vi "background writer.vi"(1 "command queue":refnum<k33>, 2 "response from processor":refnum<k33>, 3 "output type order":T6[](array[typedef]), 5 "dictionary":T4, 7 "Ring Buffer":T1, 9 "cache allocation":T5, 11 "Logging Configuration":T2={"logging path"=path "", "backup directory"=path "", "group name"="", "scans per write"=20, "has enable channel"=FALSE, "enable channel (bool)"=0, "has trigger channel"=FALSE, "trigger channel (bool)"=0, "Blocks to log"=0, "Pre-trigger samples?"=FALSE, "Edge Direction"=enum."Rising", "LogRotate"=refnum}) -> (15 "error out":errorcluster)   [LabVIEW 2015, in "TDMS datalogger runtime.lvclass"]
uses:
  TDMS datalogger runtime.lvclass
  <vilib>/NI/Tag Bus/tag/Data Type.ctl
  data cache.ctl
  <vilib>/NI/Tag Bus/dictionary/full data dictionary.ctl
  message to background process.ctl
  control enum.ctl
  <vilib>/NI/Tag Bus/table/data table.ctl
  response from background process.ctl
  response enum.ctl
  Logging Configuration.ctl
  <vilib>/NI/LogRotate/LogRotate.lvclass
  configuration/Edge Direction.ctl
  Ring Buffer.ctl
  writer state enum.ctl
  <vilib>/NI/Tag Bus/table/data table.lvlib
  <vilib>/NI/Tag Bus/tag/tag descriptor.lvclass
  <vilib>/NI/Tag Bus/dictionary/data dictionary.lvclass
  configuration/TDMS datalogger configuration.lvclass
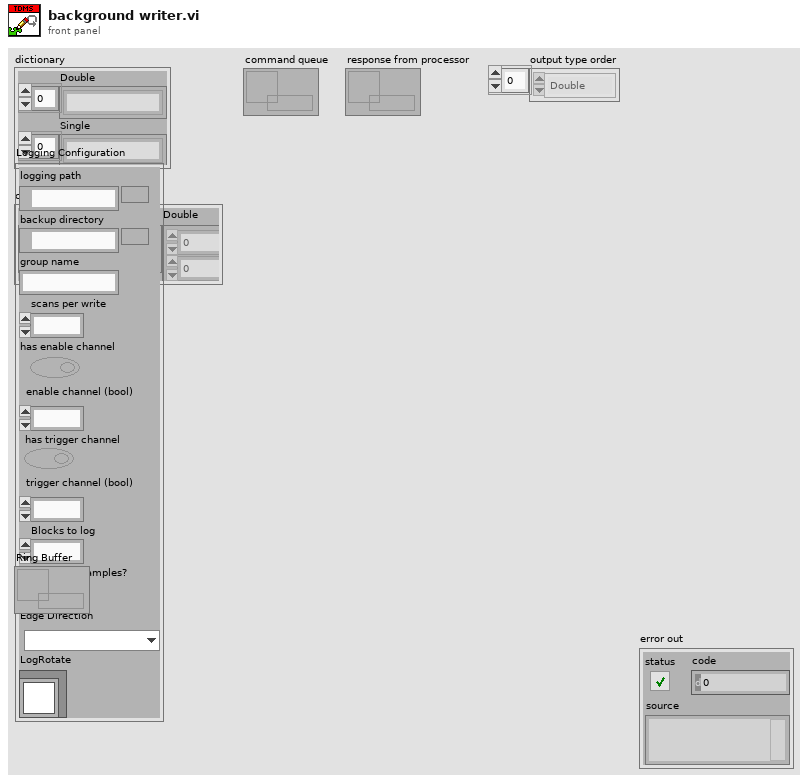
[diagram p1: front panel]
types:
  T1 = typedef "TDMS datalogger runtime.lvclass/Ring Buffer.ctl" = refnum<queue>
  T2 = typedef "TDMS datalogger runtime.lvclass/Logging Configuration.ctl" = cluster{"logging path":path, "backup directory":path, "group name":string, "scans per write":u16, "has enable channel":bool, "enable channel (bool)":i32, "has trigger channel":bool, "trigger channel (bool)":i32, "Blocks to log":i32, "Pre-trigger samples?":bool, "Edge Direction":T3, "LogRotate":refnum<class "LogRotate.lvclass">}
  T3 = typedef "TDMS datalogger configuration.lvclass/Edge Direction.ctl" = enum16{"Rising", "Falling"}
  T4 = typedef "tag bus.lvlib/data dictionary.lvclass/full data dictionary.ctl" = cluster{"Double":string[], "Single":string[], "I64":string[], "I32":string[], "I16":string[], "I8":string[], "U64":string[], "U32":string[], "U16":string[], "U8":string[], "Boolean":string[], "String":string[], "Array of Double":string[], "Array of Single":string[], "Array of I64":string[], "Array of I32":string[], "Array of I16":string[], "Array of I8":string[], "Array of U64":string[], "Array of U32":string[], "Array of U16":string[], "Array of U8":string[], "Array of Boolean":string[], "Array of String":string[]}
  T5 = typedef "TDMS datalogger runtime.lvclass/data cache.ctl" = cluster{"timestamps":timestamp[], "Double":dbl[][], "Single":sgl[][], "I64":i64[][], "I32":i32[][], "I16":i16[][], "I8":i8[][], "U64":u64[][], "U32":u32[][], "U16":u16[][], "U8":u8[][], "Boolean":bool[][]}
  T6 = typedef "tag bus.lvlib/tag descriptor.lvclass/Data Type.ctl" = enum16{"Double", "Single", "I64", "I32", "I16", "I8", "U64", "U32", "U16", "U8", "Boolean", "String", "Array of Double", "Array of Single", "Array of I64", "Array of I32", "Array of I16", "Array of I8", "Array of U64", "Array of U32", "Array of U16", "Array of U8", "Array of Boolean", "Array of String"}
  T7 = typedef "TDMS datalogger runtime.lvclass/writer state enum.ctl" = enum16{"wait for message", "create file", "report error", "exit", "close file"}
  T8 = typedef "TDMS datalogger runtime.lvclass/response enum.ctl" = enum16{"exit", "return buffer", "error"}
  T9 = typedef "TDMS datalogger runtime.lvclass/response from background process.ctl" = cluster{"response enum":T8, "datapack":refnum<data-value>, "error code":i32}
  T10 = typedef "TDMS datalogger runtime.lvclass/message to background process.ctl" = cluster{"control enum":T11, "datapack":refnum<data-value>, "Time Stamp":timestamp}
  T11 = typedef "TDMS datalogger runtime.lvclass/control enum.ctl" = enum16{"exit", "output data"}
  T12 = typedef "tag bus.lvlib/data table.lvlib/data table.ctl" = cluster{"Double":dbl[], "Single":sgl[], "I64":i64[], "I32":i32[], "I16":i16[], "I8":i8[], "U64":u64[], "U32":u32[], "U16":u16[], "U8":u8[], "Boolean":bool[], "String":string[], "Array of Double":cluster{"DBL Array":dbl[]}[], "Array of Single":cluster{"SGL Array":sgl[]}[], "Array of I64":cluster{"I64 Array":i64[]}[], "Array of I32":cluster{"I32 Array":i32[]}[], "Array of I16":cluster{"I16 Array":i16[]}[], "Array of I8":cluster{"I8 Array":i8[]}[], "Array of U64":cluster{"U64 Array":u64[]}[], "Array of U32":cluster{"U32 Array":u32[]}[], "Array of U16":cluster{"U16 Array":u16[]}[], "Array of U8":cluster{"U8 Array":u8[]}[], "Array of Boolean":cluster{"Boolean Array":bool[]}[], "Array of String":cluster{"String Array":string[]}[]}
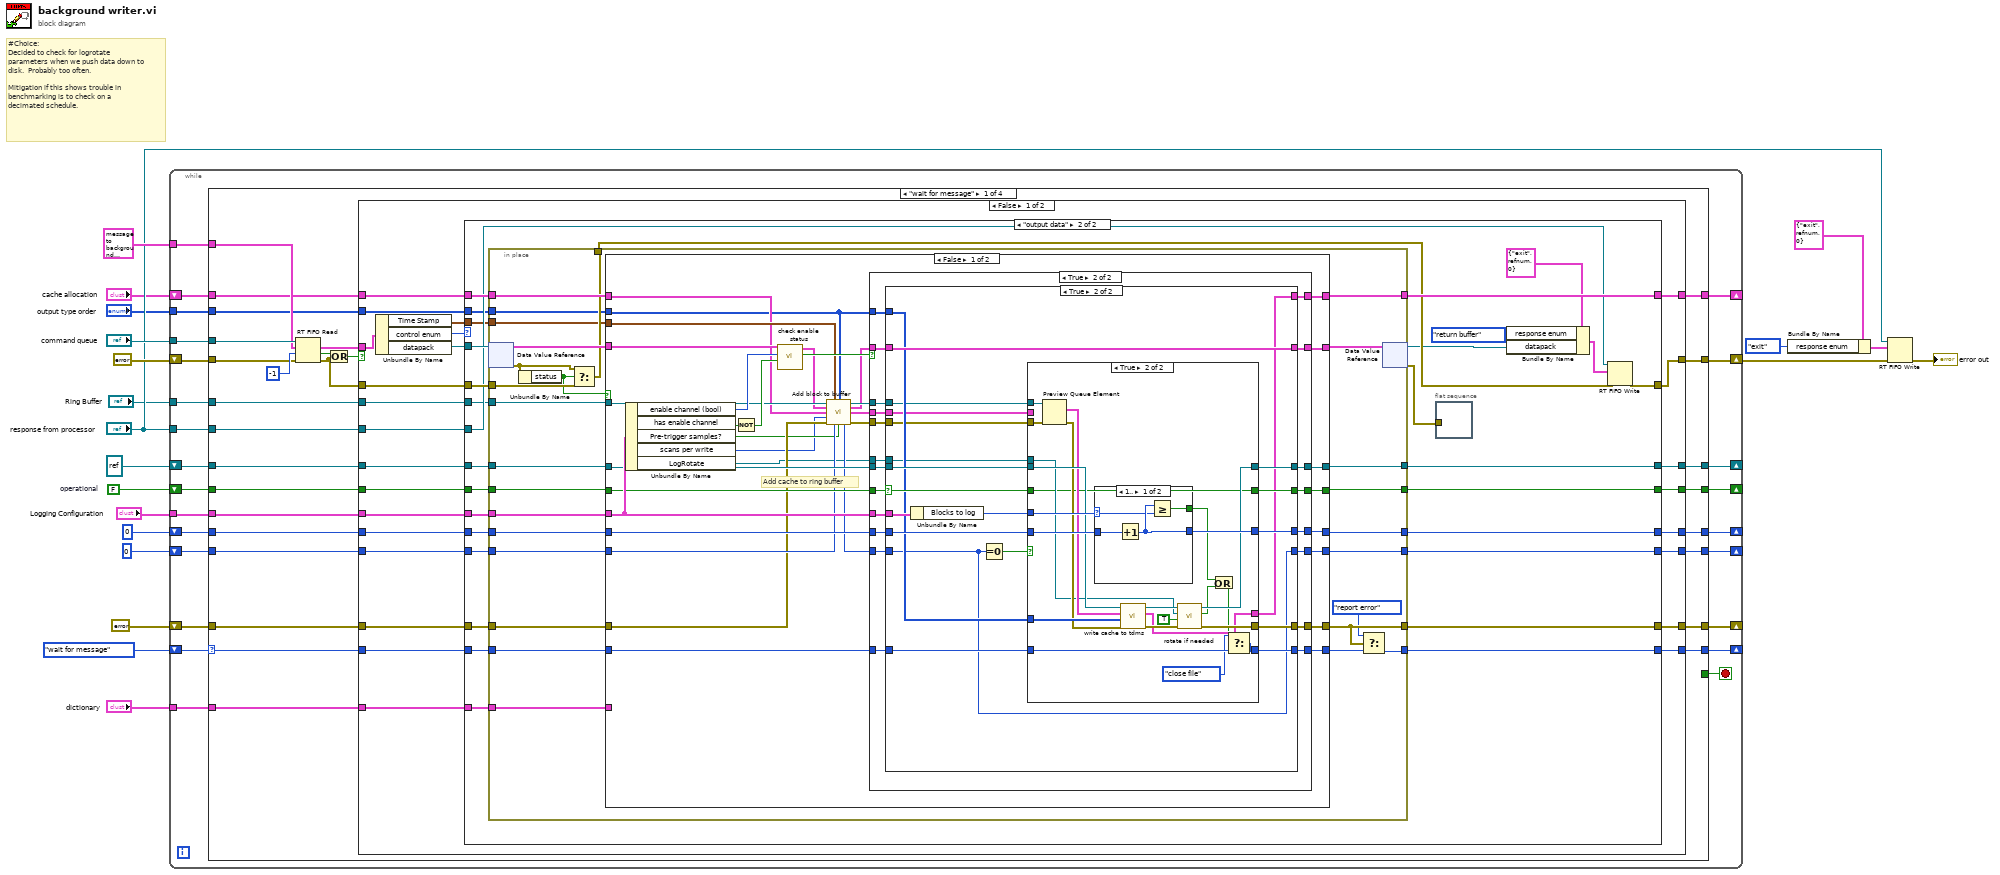
[diagram p0: block diagram]
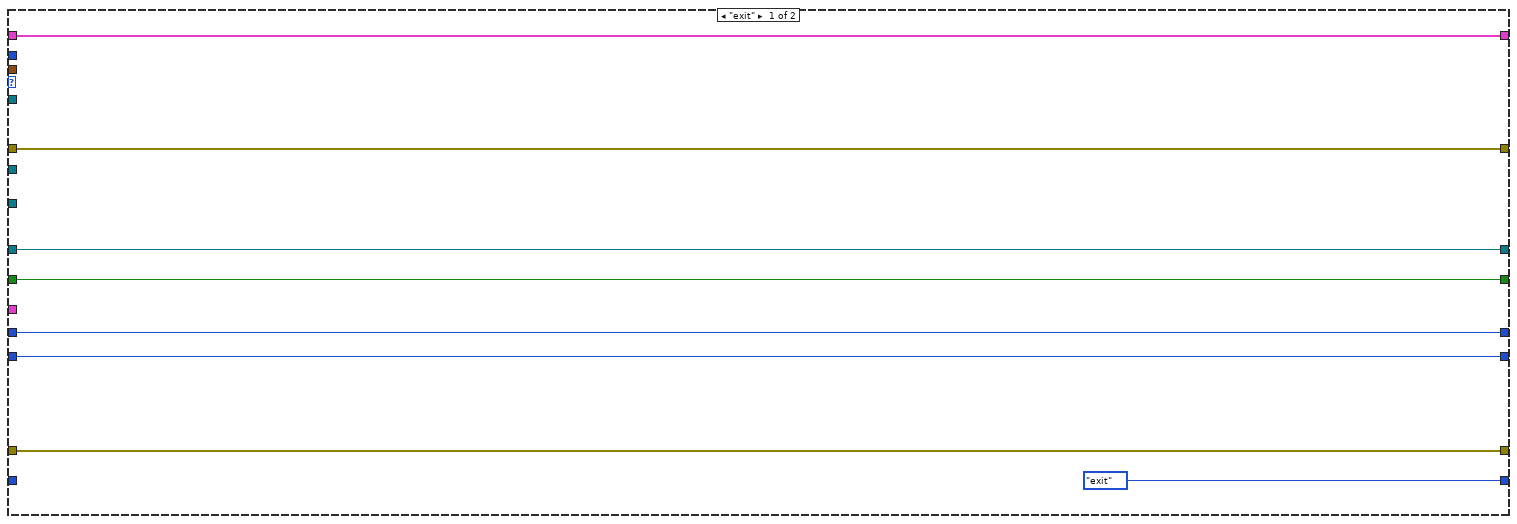
[diagram p2: hidden frame]
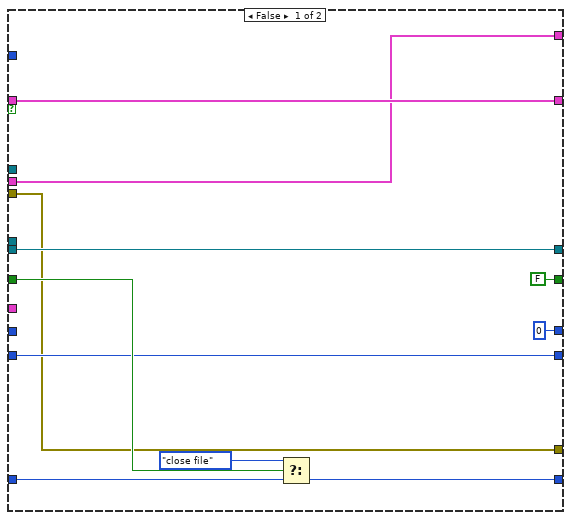
[diagram p3: hidden frame]
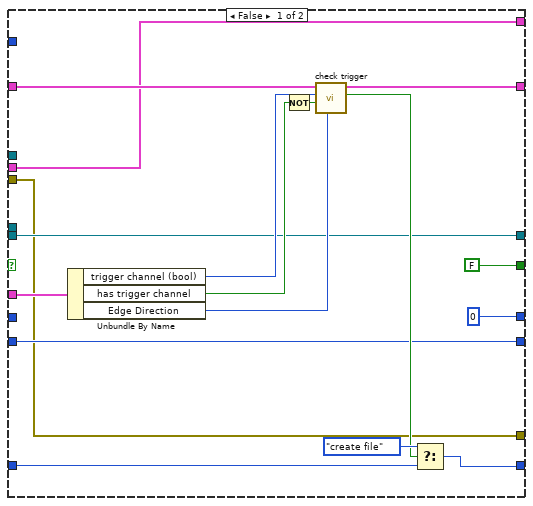
[diagram p4: hidden frame]
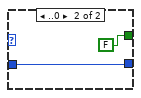
[diagram p6: hidden frame]
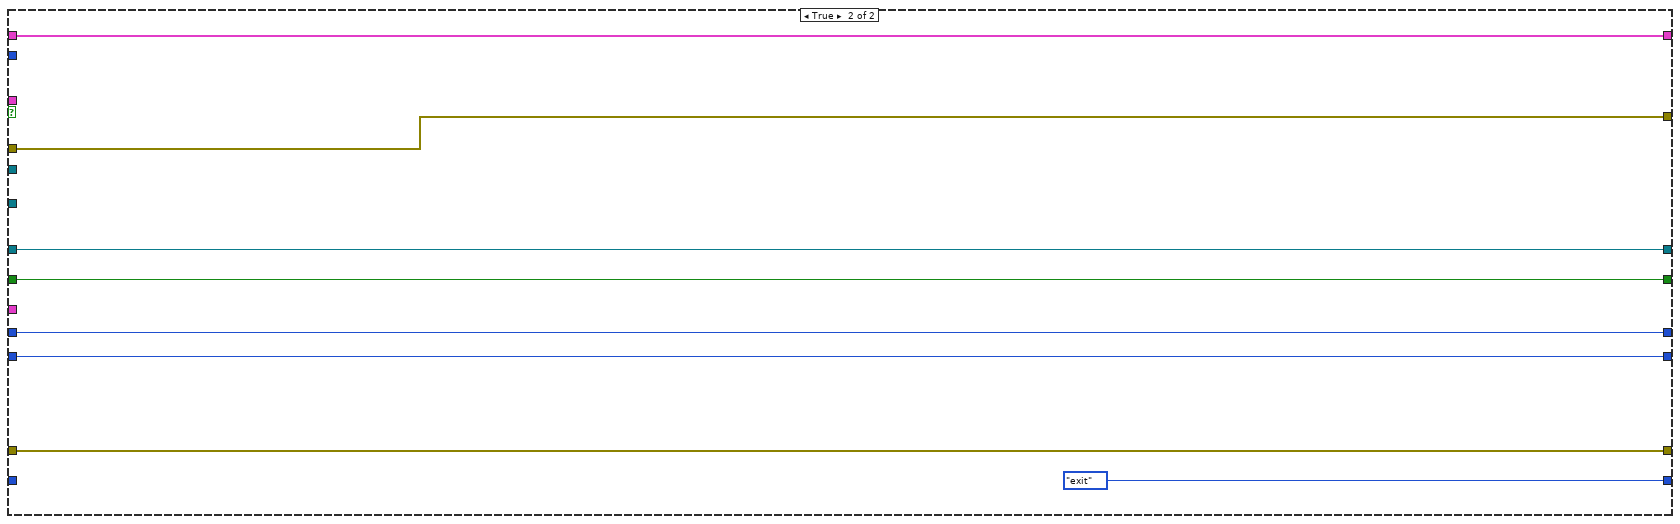
[diagram p8: hidden frame]
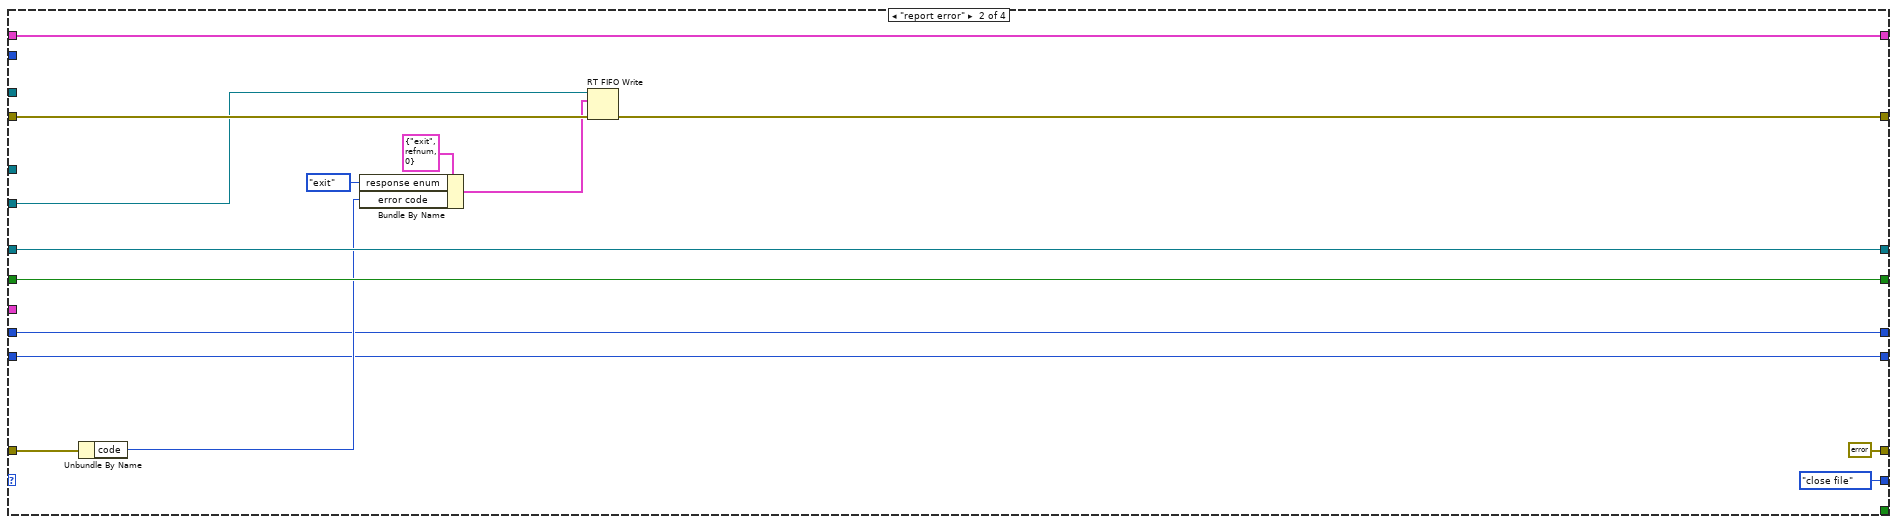
[diagram p9: hidden frame]
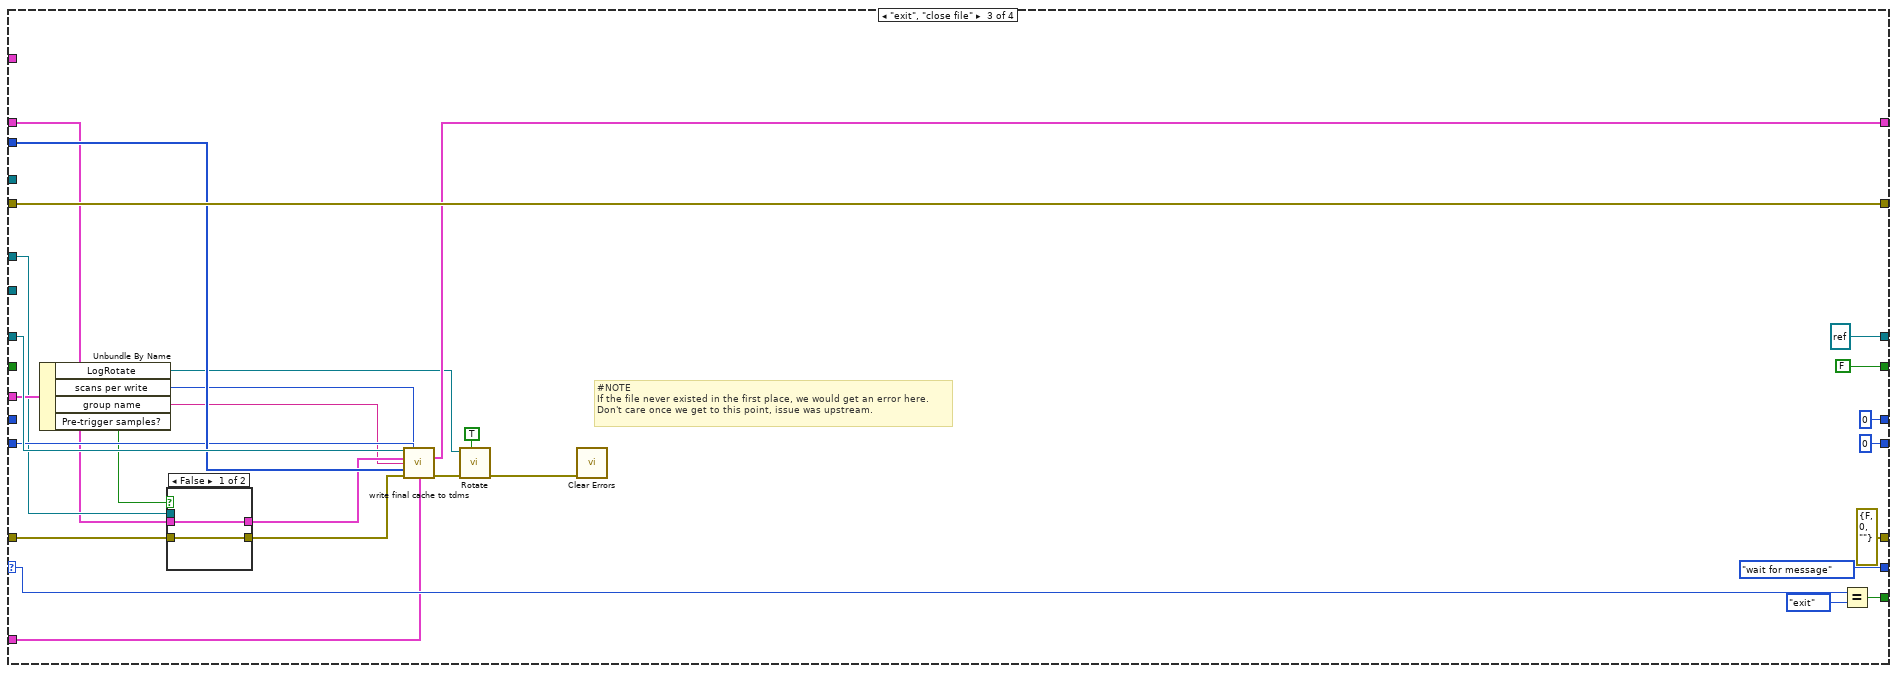
[diagram p10: hidden frame]
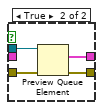
[diagram p11: hidden frame]
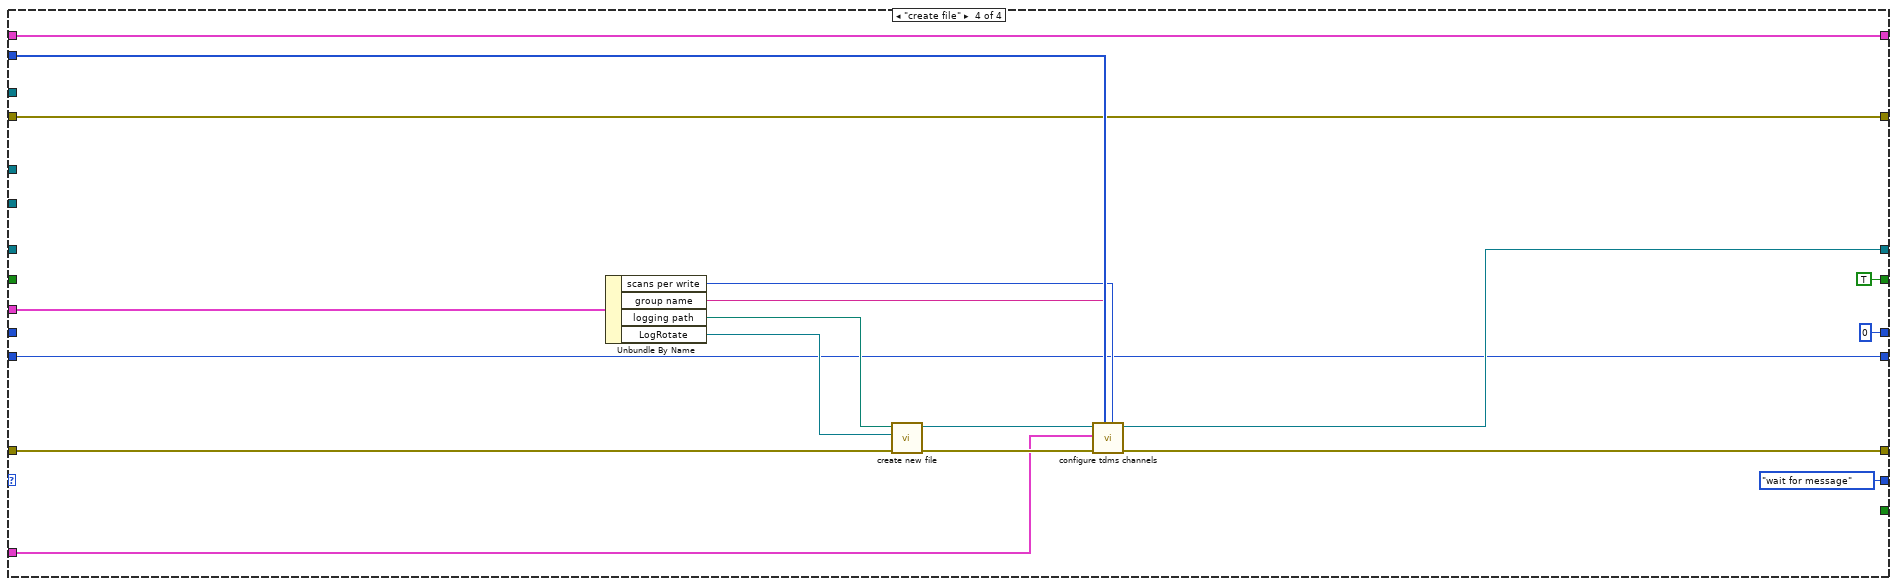
[diagram p12: hidden frame]
diagram:
  w9 = FALSE  # operational
  # "#Choice:\nDecided to check for logrotate parameters when we push data down to disk.  Probably too often.\n\nMitigation if this shows trouble in benchmarking is to check on a decimated schedule."
  n1 = while {
    tunnel: "command queue" -> [w44]
    tunnel: T10 {"control enum"=enum."exit", "datapack"=refnum, "Time Stamp"=timestamp(0 s since 1904-01-01)} ("element") -> [w43]
    shift-right: [w41] -> w17
    shift-left: errorcluster {"status"=FALSE, "code"=0, "source"=""} ("error in") -> [w42]
    tunnel: "response from processor" -> [w39]
    shift-right: [w37] -> _
    shift-left: writer_state_enum."wait for message" ("logger state") -> [w38]
    shift-right: [w35] -> _
    shift-left: refnum<k34> refnum ("tdms file out") -> [w36]
    shift-right: [w29] -> _
    shift-left: w9 -> [w34]
    shift-right: [w32] -> _
    shift-left: errorcluster {"status"=FALSE, "code"=0, "source"=""} ("error in") -> [w33]
    tunnel: "dictionary" -> [w31]
    tunnel: "output type order" -> [w30]
    shift-right: [w28] -> _
    shift-left: 0 ("sample counter") -> [w27]
    shift-right: [w25] -> _
    shift-left: "cache allocation" -> [w26]
    shift-right: [w24] -> _
    shift-left: u16 0 ("Blocks written out") -> [w23]
    tunnel: "Ring Buffer" -> [w22]
    tunnel: "Logging Configuration" -> [w21]
    stop <- w40 stop-if-true
    n2 = case shown="\"wait for message\"" w38 {
      selector: w38 -> [w51 _ w354 _]
      tunnel: w44 -> [w72 _ _ _]
      tunnel: w43 -> [w70 _ _ _]
      tunnel: w42 -> [w69 w328 w356 w363]
      tunnel: [w65 w326 w356 w363] -> w41
      tunnel: [_ _ w355 _] -> w40
      tunnel: w39 -> [w63 w325 _ _]
      tunnel: [w62 writer_state_enum."close file" ("logger state") writer_state_enum."wait for message" ("logger state") writer_state_enum."wait for message" ("logger state")] -> w37
      tunnel: w36 -> [w61 w327 w348 _]
      tunnel: [w60 w327 refnum<k34> refnum ("tdms file out") w369] -> w35
      tunnel: w34 -> [w58 w319 _ _]
      tunnel: w33 -> [w56 w318 w336 w380]
      tunnel: [w57 errorcluster {"status"=FALSE, "code"=0, "source"=""} ("error out") errorcluster {"status"=FALSE, "code"=0, "source"=""} ("error out") w370] -> w32
      tunnel: w31 -> [w49 _ w345 w378]
      tunnel: w30 -> [w50 _ w347 w377]
      tunnel: [w59 w319 FALSE TRUE ("operational")] -> w29
      tunnel: [w54 w315 0 ("sample counter") w366] -> w28
      tunnel: w27 -> [w55 w315 w346 w366]
      tunnel: w26 -> [w53 w316 w332 w364]
      tunnel: [w52 w316 w344 w364] -> w25
      tunnel: [w48 w314 u16 0 ("Blocks written out") u16 0 ("Blocks written out")] -> w24
      tunnel: w23 -> [w47 w314 _ _]
      tunnel: w22 -> [w46 _ w334 _]
      tunnel: w21 -> [w45 _ w338 w376]
      frame "wait for message" {
        n3 = RT FIFO Read(0:w72, 1:w70, 2:-1 ("timeout in ms (0)"), 3:w69) -> (9:w64:T10, 10:w68:bool, 11:w66:errorcluster)  [unwired: 2 out]
        n4 = Or(x=w68, y=w66) -> (x .or. y?=w67:bool)
        n5 = case shown="False" w67 {
          tunnel: w66 -> [w94 w313]
          tunnel: [w95 w313] -> w65
          tunnel: w64 -> [w97 _]
          tunnel: w63 -> [w92 _]
          tunnel: [w91 writer_state_enum."exit" ("logger state")] -> w62
          tunnel: w61 -> [w90 w311]
          tunnel: [w89 w311] -> w60
          tunnel: [w87 w310] -> w59
          tunnel: w58 -> [w88 w310]
          tunnel: [w86 w309] -> w57
          tunnel: w56 -> [w85 w309]
          tunnel: w55 -> [w83 w308]
          tunnel: [w84 w308] -> w54
          tunnel: w53 -> [w82 w307]
          tunnel: [w81 w307] -> w52
          tunnel: w51 -> [w80 _]
          tunnel: w50 -> [w79 _]
          tunnel: w49 -> [w78 _]
          tunnel: [w77 w306] -> w48
          tunnel: w47 -> [w76 w306]
          tunnel: w46 -> [w75 _]
          tunnel: w45 -> [w74 _]
          frame False {
            n6 = Unbundle By Name(w97) -> ("Time Stamp"=w73:timestamp, "control enum"=w96:T11, "datapack"=w93:refnum<data-value>)
            n7 = case shown="\"output data\"" w96 {
              tunnel: [w105 w120] -> w95
              tunnel: w94 -> [w105 w133]
              tunnel: w93 -> [_ w134]
              tunnel: w92 -> [_ w117]
              tunnel: [writer_state_enum."exit" ("logger state") w122] -> w91
              tunnel: w90 -> [w103 w132]
              tunnel: [w103 w131] -> w89
              tunnel: w88 -> [w102 w129]
              tunnel: [w102 w130] -> w87
              tunnel: [w101 w123] -> w86
              tunnel: w85 -> [w101 w124]
              tunnel: [w99 w127] -> w84
              tunnel: w83 -> [w99 w128]
              tunnel: w82 -> [w100 w125]
              tunnel: [w100 w126] -> w81
              tunnel: w80 -> [_ w121]
              tunnel: w79 -> [_ w112]
              tunnel: w78 -> [_ w111]
              tunnel: [w98 w110] -> w77
              tunnel: w76 -> [w98 w109]
              tunnel: w75 -> [_ w108]
              tunnel: w74 -> [_ w107]
              tunnel: w73 -> [_ w106]
              frame "exit" {
              }
              frame "output data" {
                n8 = in-place {
                  in-place-border: w133 -> [w161]
                  in-place-border: w132 -> [w156]
                  in-place-border: [w155] -> w131
                  in-place-border: [w154] -> w130
                  in-place-border: w129 -> [w153]
                  in-place-border: w128 -> [w152]
                  in-place-border: [w151] -> w127
                  in-place-border: [w150] -> w126
                  in-place-border: w125 -> [w149]
                  in-place-border: w124 -> [w148]
                  in-place-border: [w138] -> w123
                  in-place-border: [w135] -> w122
                  in-place-border: w121 -> [w147]
                  in-place-border: [w146] -> w119
                  in-place-border: w112 -> [w145]
                  in-place-border: w111 -> [w144]
                  in-place-border: [w143] -> w110
                  in-place-border: w109 -> [w142]
                  in-place-border: w108 -> [w141]
                  in-place-border: w107 -> [w140]
                  in-place-border: w106 -> [w139]
                  n9 = in-place-dvr #1(w134) -> (w157:T12, w160:errorcluster)
                  n10 = Unbundle By Name(w160) -> ("status"=w159:bool)
                  n11 = Select(t=w160, s=w159, f=w161) -> (s? t:f=w146:errorcluster)
                  n12 = case shown="False" w159 {
                    tunnel: [w194 w305] -> w158
                    tunnel: w157 -> [w174 w305]
                    tunnel: w156 -> [w183 w304]
                    tunnel: [w182 w304] -> w155
                    tunnel: [w185 w303] -> w154
                    tunnel: w153 -> [w189 w303]
                    tunnel: w152 -> [w173 w302]
                    tunnel: [w184 w302] -> w151
                    tunnel: [w181 w301] -> w150
                    tunnel: w149 -> [w167 w301]
                    tunnel: w148 -> [w170 w300]
                    tunnel: [w191 w300] -> w138
                    tunnel: [w192 w299] -> w137
                    tunnel: w147 -> [w193 w299]
                    tunnel: w145 -> [w162 _]
                    tunnel: w144 -> [_ _]
                    tunnel: [w186 w298] -> w143
                    tunnel: w142 -> [w187 w298]
                    tunnel: w141 -> [w175 _]
                    tunnel: w140 -> [w190 _]
                    tunnel: w139 -> [w171 _]
                    frame False {
                      # "Add cache to ring buffer"
                      n13 = Unbundle By Name(w190) -> ("enable channel (bool)"=w180:i32, "has enable channel"=w179:bool, "Pre-trigger samples?"=w165:bool, "scans per write"=w163:u16, "LogRotate"=w164:refnum<class "LogRotate.lvclass">)
                      n14 = Not(x=w179) -> (.not. x?=w178:bool)
                      n15 = call "check enable status.vi"("always enabled?"=w178, "enable channel index"=w180, "data table in"=w174) -> ("enabled?"=w188:bool, "Data table out"=w169:T12)  [unwired: 7 in]
                      n16 = call "Add block to buffer.vi"("Ring Buffer"=w175, "Time Stamp"=w171, "output type order"=w162, "data table in"=w169, "cache in"=w167, "Block size"=w163, "error in (no error)"=w170, "sample counter in"=w173, "Pre-trigger samples?"=w165) -> ("Ring Buffer out"=w177:T1, "data table out"=w168:T12, "cache out"=w166:T5, "Sample counter out"=w172:i32, "error out"=w176:errorcluster)  [unwired: 2 in]
                      n17 = case shown="True" w188 {
                        tunnel: [w201 w225] -> w194
                        tunnel: w193 -> [w204 w224]
                        tunnel: [w202 w223] -> w192
                        tunnel: [w196 w207] -> w191
                        tunnel: w190 -> [_ w222]
                        tunnel: w168 -> [w201 w221]
                        tunnel: w189 -> [w205 w220]
                        tunnel: w172 -> [w199 w219]
                        tunnel: w187 -> [_ w218]
                        tunnel: [u16 0 ("Blocks written out") w217] -> w186
                        tunnel: [FALSE w216] -> w185
                        tunnel: [w199 w215] -> w184
                        tunnel: w183 -> [w197 w214]
                        tunnel: [w197 w213] -> w182
                        tunnel: w162 -> [_ w212]
                        tunnel: [w195 w211] -> w181
                        tunnel: w177 -> [_ w210]
                        tunnel: w176 -> [w196 w209]
                        tunnel: w166 -> [w195 w208]
                        tunnel: w164 -> [_ w206]
                        frame False {
                          n18 = Select(t=writer_state_enum."close file", s=w205, f=w204) -> (s? t:f=w202:T7)
                        }
                        frame True {
                          n19 = case shown="True" w220 {
                            selector: w220 -> [_ w257]
                            tunnel: w221 -> [w232 w255]
                            tunnel: [w242 w255] -> w225
                            tunnel: w224 -> [w241 w245]
                            tunnel: [w239 w244] -> w223
                            tunnel: w222 -> [w238 w262]
                            tunnel: w219 -> [w231 w243]
                            tunnel: w218 -> [_ w261]
                            tunnel: [u16 0 ("Blocks written out") w259] -> w217
                            tunnel: [FALSE w258] -> w216
                            tunnel: [w231 w243] -> w215
                            tunnel: w214 -> [w228 w254]
                            tunnel: [w228 w253] -> w213
                            tunnel: w212 -> [_ w252]
                            tunnel: [w227 w251] -> w211
                            tunnel: w210 -> [_ w250]
                            tunnel: w209 -> [w226 w248]
                            tunnel: w208 -> [w227 w247]
                            tunnel: [w226 w256] -> w207
                            tunnel: w206 -> [_ w249]
                            frame False {
                              n20 = Unbundle By Name(w238) -> ("trigger channel (bool)"=w237:i32, "has trigger channel"=w236:bool, "Edge Direction"=w234:T3)
                              n21 = Not(x=w236) -> (.not. x?=w235:bool)
                              n22 = call "check trigger.vi"("Edge Direction"=w234, "No trigger?"=w235, "triggerchannel index"=w237, "data table in"=w232) -> ("Trigger"=w233:bool, "Data table out"=w242:T12)  [unwired: 6 in]
                              n23 = Select(t=writer_state_enum."create file", s=w233, f=w241) -> (s? t:f=w239:T7)
                            }
                            frame True {
                              n24 = Unbundle By Name(w262) -> ("Blocks to log"=w260:i32)
                              n25 = Equal To 0?(x=w243) -> (x = 0?=w246:bool)
                              n26 = case shown="True" w246 {
                                tunnel: w261 -> [w267 w291]
                                tunnel: w260 -> [_ w290]
                                tunnel: [w267 w287] -> w259
                                tunnel: [w268 w275] -> w258
                                tunnel: w257 -> [w268 w275]
                                tunnel: [w264 w286] -> w256
                                tunnel: w254 -> [w266 w285]
                                tunnel: [w266 w284] -> w253
                                tunnel: w252 -> [_ w283]
                                tunnel: [w265 w281] -> w251
                                tunnel: w250 -> [_ w280]
                                tunnel: w249 -> [_ w276]
                                tunnel: w248 -> [w264 w279]
                                tunnel: w247 -> [w265 _]
                                tunnel: w245 -> [w263 w274]
                                tunnel: [w263 w269] -> w244
                                frame False {
                                }
                                frame True {
                                n27 = Preview Queue Element(queue=w280, error in (no error)=w279) -> (element=w278:T5, error out=w277:errorcluster)  [unwired: 1 in, 2 out]
                                n28 = case shown="1.." w290 {
                                selector: w290 -> [w292 _]
                                tunnel: w291 -> [w295 w297]
                                tunnel: [w293 w297] -> w287
                                tunnel: [w294 FALSE] -> w273
                                frame 1.. {
                                n29 = Increment(x=w295) -> (x+1=w293:u16)
                                n30 = Greater Or Equal?(x=w293, y=w292) -> (x >= y?=w294:bool)
                                }
                                frame ..0 {
                                }
                                }
                                n31 = call "write cache to tdms.vi"("error in"=w277, "output type order"=w283, "cache in"=w278, "tdms file in"=w285) -> ("error out"=w289:errorcluster, "cache out"=w281:T5, "tdms file out"=w288:refnum<k34>)  [unwired: 5 in]
                                n32 = call "rotate if needed.vi"("error in"=w289, "Check?"=TRUE, "LogRotate"=w276, "tdms ref in"=w288) -> ("error out"=w286:errorcluster, "rotated?"=w272:bool, "tdms ref out"=w284:refnum<k34>)  [unwired: 5 in]
                                n33 = Or(x=w273, y=w272) -> (x .or. y?=w270:bool)
                                n34 = Select(t=writer_state_enum."close file", s=w270, f=w274) -> (s? t:f=w269:T7)
                                }
                              }
                            }
                          }
                        }
                      }
                    }
                    frame True {
                    }
                  }
                  n35 = Select(t=writer_state_enum."report error", s=w138, f=w137) -> (s? t:f=w135:T7)
                  n36 = in-place-dvr #1(w158) -> (w114:refnum<data-value>, w118:errorcluster)
                }
                n37 = flat-sequence {
                  tunnel: w118 -> [_]
                  frame #0 {
                  }
                }
                n38 = Bundle By Name(cluster=T9 {"response enum"=enum."exit", "datapack"=refnum, "error code"=0} ("element"), "response enum"=response_enum."return buffer", "datapack"=w114) -> (w115:T9)
                n39 = RT FIFO Write(0:w117, 1:w115, 3:w119) -> (11:w120:errorcluster)  [unwired: 2 in, 3 out]
              }
            }
          }
          frame True {
          }
        }
      }
      frame "report error" {
        n40 = Unbundle By Name(w318) -> ("code"=w317:i32)
        n41 = Bundle By Name(cluster=T9 {"response enum"=enum."exit", "datapack"=refnum, "error code"=0} ("element"), "response enum"=response_enum."exit", "error code"=w317) -> (w323:T9)
        n42 = RT FIFO Write(0:w325, 1:w323, 3:w328) -> (11:w326:errorcluster)  [unwired: 2 in, 3 out]
      }
      frame "exit", "close file" {
        # "#NOTE\nIf the file never existed in the first place, we would get an error here.\nDon't care once we get to this point, issue was upstream."
        n43 = Unbundle By Name(w338) -> ("LogRotate"=w339:refnum<class "LogRotate.lvclass">, "scans per write"=w331:u16, "group name"=w330:string, "Pre-trigger samples?"=w329:bool)
        n44 = case shown="False" w329 {
          tunnel: w336 -> [w358 w362]
          tunnel: [w358 w361] -> w335
          tunnel: w334 -> [_ w360]
          tunnel: [w357 w359] -> w333
          tunnel: w332 -> [w357 _]
          frame False {
          }
          frame True {
            n45 = Preview Queue Element(queue=w360, error in (no error)=w362) -> (element=w359:T5, error out=w361:errorcluster)  [unwired: 1 in, 2 out]
          }
        }
        n46 = call "write final cache to tdms.vi"("tdms file in"=w348, "sample counter"=w346, "cache in"=w333, "group name"=w330, "output type order"=w347, "error in"=w335, "scans per write"=w331, "dictionary"=w345) -> ("cache out"=w344:T5, "error out"=w341:errorcluster)  [unwired: 6 in]
        n47 = call <vilib>:"Rotate.vi"("Force rotate"=TRUE, "error in (no error)"=w341, "LogRotate in"=w339) -> ("error out"=w343:errorcluster)  [unwired: 7 in, 1 out]
        n48 = call <vilib>:"Clear Errors.vi"("error in (no error)"=w343) -> ()  [unwired: 5 in, 2 out]
        n49 = Equal?(x=w354, y=writer_state_enum."exit") -> (x = y?=w355:bool)
      }
      frame "create file" {
        n50 = Unbundle By Name(w376) -> ("scans per write"=w371:u16, "group name"=w372:string, "logging path"=w375:path, "LogRotate"=w374:refnum<class "LogRotate.lvclass">)
        n51 = call "create new file.vi"("error in"=w380, "LogRotate in"=w374, "logging path"=w375) -> ("error out"=w379:errorcluster, "tdms file out"=w373:refnum<k34>)  [unwired: 7 in]
        n52 = call "configure tdms channels.vi"("samples per channel (1)"=w371, "type order"=w377, "group name"=w372, "error in"=w379, "dictionary"=w378, "tdms file in"=w373) -> ("error out"=w370:errorcluster, "tdms file out"=w369:refnum<k34>)  [unwired: 4 in]
      }
    }
  }
  n53 = Bundle By Name(cluster=T9 {"response enum"=enum."exit", "datapack"=refnum, "error code"=0} ("element"), "response enum"=response_enum."exit") -> (w14:T9)
  n54 = RT FIFO Write(0:"response from processor", 1:w14, 3:w17) -> (11:→"error out":errorcluster)  [unwired: 2 in, 3 out]
